vi "assign data to cluster (SubVI).vi"(9 "Inv1 high speed DAQ \nsignal scaling control":T3, 10 "sampling rate (Hz)":i32, 11 "Data":T1) -> (3 "Raw Data":T2)   [LabVIEW 2019, in "Main.lvclass"]
doc: "Developed by Kevin Thompson\nkevin@thompsonengineering.net\n\nCopyright 2020\nThompson Engineering, LLC"
uses:
  Main.lvclass
  DataTypes/Gain control.ctl
  DataTypes/raw data variables.ctl
  DataTypes/data queue typedef.ctl
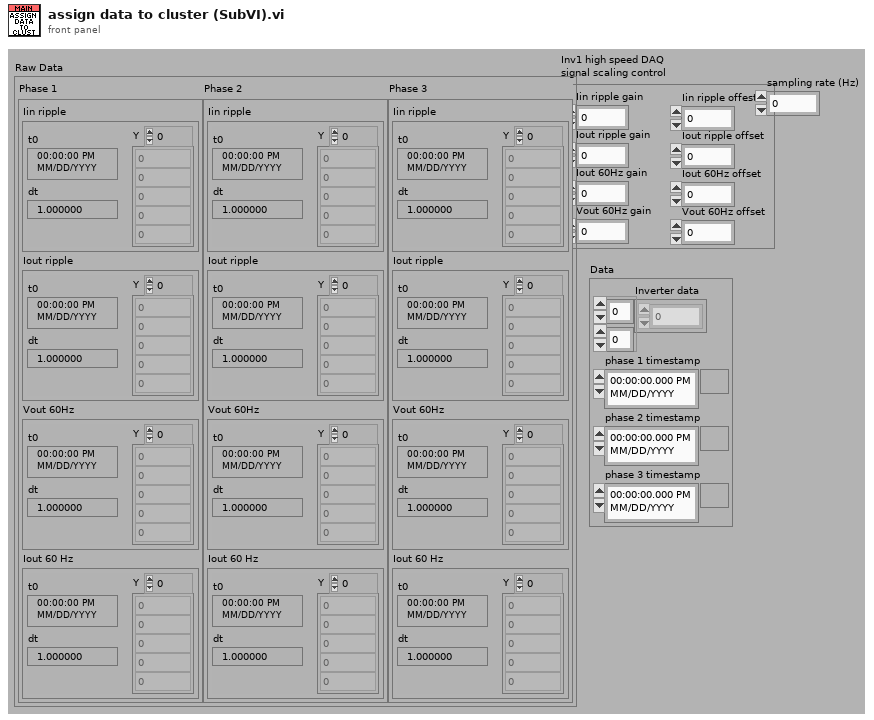
[diagram p1: front panel]
types:
  T1 = typedef "Main.lvclass/data queue typedef.ctl" = cluster{"Inverter data":dbl[][], "phase 1 timestamp":timestamp, "phase 2 timestamp":timestamp, "phase 3 timestamp":timestamp}
  T2 = typedef "Main.lvclass/raw data variables.ctl" = cluster{"Phase 1":cluster{"Iin ripple":waveform(dbl), "Iout ripple":waveform(dbl), "Vout 60Hz":waveform(dbl), "Iout 60 Hz":waveform(dbl)}, "Phase 2":cluster{"Iin ripple":waveform(dbl), "Iout ripple":waveform(dbl), "Vout 60Hz":waveform(dbl), "Iout 60 Hz":waveform(dbl)}, "Phase 3":cluster{"Iin ripple":waveform(dbl), "Iout ripple":waveform(dbl), "Vout 60Hz":waveform(dbl), "Iout 60 Hz":waveform(dbl)}}
  T3 = typedef "Main.lvclass/Gain control.ctl" = cluster{"Iin ripple gain":dbl, "Iout ripple gain":dbl, "Iout 60Hz gain ":dbl, "Vout 60Hz gain ":dbl, "Iin ripple offest":dbl, "Iout ripple offset":dbl, "Iout 60Hz offset":dbl, "Vout 60Hz offset":dbl}
  T4 = cluster{"ch0":waveform(dbl), "ch1":waveform(dbl), "ch2":waveform(dbl), "ch3":waveform(dbl)}
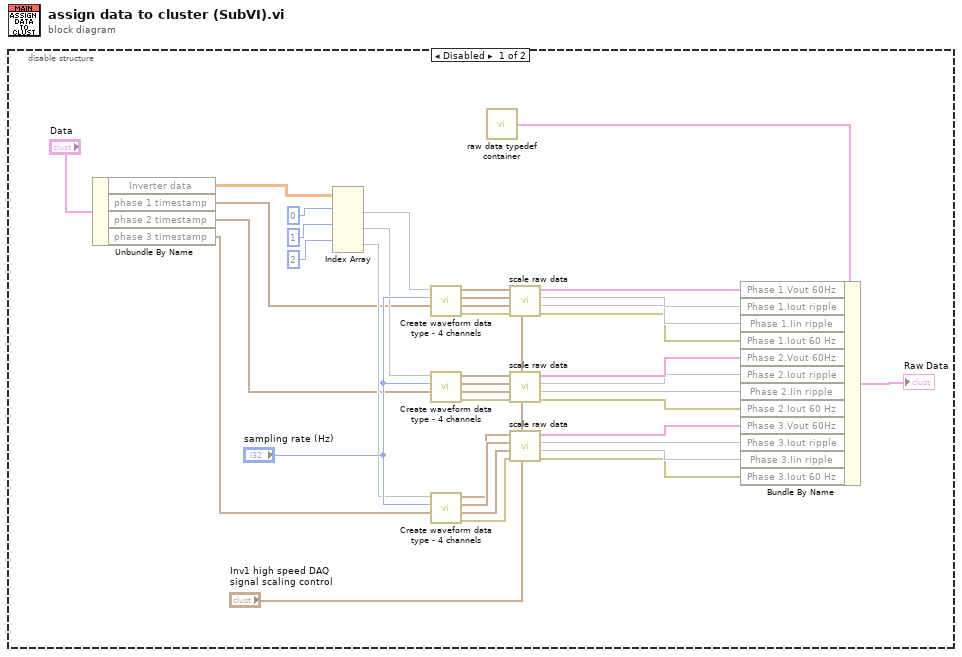
[diagram p0: block diagram]
diagram:
  n1 = disable-structure shown="Disabled" {
    frame Disabled {
      n2 = Unbundle By Name("Data") -> ("Inverter data"=w5:dbl[][], "phase 1 timestamp"=w4:timestamp, "phase 2 timestamp"=w3:timestamp, "phase 3 timestamp"=w2:timestamp)
      n3 = Index Array(array=w5, index (row) #1=0 ("disabled index (col)"), index (row) #2=1 ("index (col)"), index (row) #3=2 ("index (col)")) -> (element #1=w7:dbl[], element #2=w8:dbl[], element #3=w9:dbl[])  [unwired: 3 in]
      n4 = call "raw data typedef container.vi"() -> ("Acquired Data"=w23:T2)
      n5 = call "Create waveform data type - 4 channels.vi"(3:w32, "Time Stamp"=w4, "sampling rate (Hz)"="sampling rate (Hz)", "scan data"=w7) -> ("error out"=w35:errorcluster, "Channel 3"=w34:waveform(dbl), "Channel 2"=w33:waveform(dbl))  [unwired: 3 in, 2 out]
      n6 = call "scale raw data.vi"("ch3"="Inv1 high speed DAQ \nsignal scaling control", "error in (no error)"=w35, "ch2"=w34, "ch1"=w33) -> ("error out"=w24:errorcluster, 1:w25, 2:w26, "output channels WF"=w1:T4, "ch0"=w32:waveform(dbl))  [unwired: 2 in, 1 out]
      n7 = call "Create waveform data type - 4 channels.vi"(3:w29, "Time Stamp"=w3, "sampling rate (Hz)"="sampling rate (Hz)", "scan data"=w8) -> ("error out"=w10:errorcluster, "Channel 3"=w31:waveform(dbl), "Channel 2"=w30:waveform(dbl))  [unwired: 3 in, 2 out]
      n8 = call "scale raw data.vi"("ch3"="Inv1 high speed DAQ \nsignal scaling control", "error in (no error)"=w10, "ch2"=w31, "ch1"=w30) -> ("error out"=w19:errorcluster, 1:w20, 2:w21, "output channels WF"=w22:T4, "ch0"=w29:waveform(dbl))  [unwired: 2 in, 1 out]
      n9 = call "Create waveform data type - 4 channels.vi"(3:w36, "Time Stamp"=w2, "sampling rate (Hz)"="sampling rate (Hz)", "scan data"=w9) -> ("error out"=w39:errorcluster, "Channel 3"=w38:waveform(dbl), "Channel 2"=w37:waveform(dbl))  [unwired: 3 in, 2 out]
      n10 = call "scale raw data.vi"("ch3"="Inv1 high speed DAQ \nsignal scaling control", "error in (no error)"=w39, "ch2"=w38, "ch1"=w37) -> ("error out"=w15:errorcluster, 1:w16, 2:w17, "output channels WF"=w18:T4, "ch0"=w36:waveform(dbl))  [unwired: 2 in, 1 out]
      n11 = Bundle By Name(cluster=w23, "Phase 1.Vout 60Hz"=w1, "Phase 1.Iout ripple"=w26, "Phase 1.Iin ripple"=w25, "Phase 1.Iout 60 Hz"=w24, "Phase 2.Vout 60Hz"=w22, "Phase 2.Iout ripple"=w21, "Phase 2.Iin ripple"=w20, "Phase 2.Iout 60 Hz"=w19, "Phase 3.Vout 60Hz"=w18, "Phase 3.Iout ripple"=w17, "Phase 3.Iin ripple"=w16, "Phase 3.Iout 60 Hz"=w15) -> (→"Raw Data":T2)
    }
    frame Enabled {
    }
  }
